vi "Send Cmd To Stimulator.vi"(0 "Stimulator":T1={"Stim Open Data"={"Name"="", "Mode"=enum."LIVE", "Visa Timeout"=0}, "Stim Init Data"={"Frequency"=0.0, "N Factor"=0, "D/T Int"=0.0, "Active Channels"=[FALSE], "LF Channels"=[]}, "Stim Update Data"={"Pulse Mode"=[], "Current"=[], "Pulse Dur"=[]}, "Stim Status"={"Open"=FALSE, "On"=FALSE}}, 1 "Command":T7, 3 "error in (no error)":errorcluster) -> (4 "Numeric Response":u8, 5 "Stimulator":T1={"Stim Open Data"={"Name"="", "Mode"=enum."LIVE", "Visa Timeout"=0}, "Stim Init Data"={"Frequency"=0.0, "N Factor"=0, "D/T Int"=0.0, "Active Channels"=[FALSE], "LF Channels"=[]}, "Stim Update Data"={"Pulse Mode"=[], "Current"=[], "Pulse Dur"=[]}, "Stim Status"={"Open"=FALSE, "On"=FALSE}}, 6 "Command":T7, 7 "Log Entry":string, 8 "error out":errorcluster)   [LabVIEW 2019]
uses:
  Data Type Defs/Stimulator.ctl
  Data Type Defs/Stim Open Data.ctl
  Data Type Defs/Stim Init Data.ctl
  Data Type Defs/Stim Update Data.ctl
  Data Type Defs/Pulse Mode (array).ctl
  Data Type Defs/Stim Status.ctl
  Bits Library/Get Bit (U8).vi
  Bits Library/Change Bit (U8).vi
  Bits Library/Bits.lvlib
panel:
  out "Write Error":errorcluster
  out "Bytes written":u32
  out "Bytes read":u32
  out "Read Error":errorcluster
  out "resulting string":string
  out "string":string
  out "hex integer string":string
  out "Number Out":u8 format="%.0x"
  out "appended array":bool[](array[boolean])
  out "element":u8 format="%0d"
  out "unsigned byte array 2":u8[](array[numeric]) format="%08b"
  out "Bytes available":u32
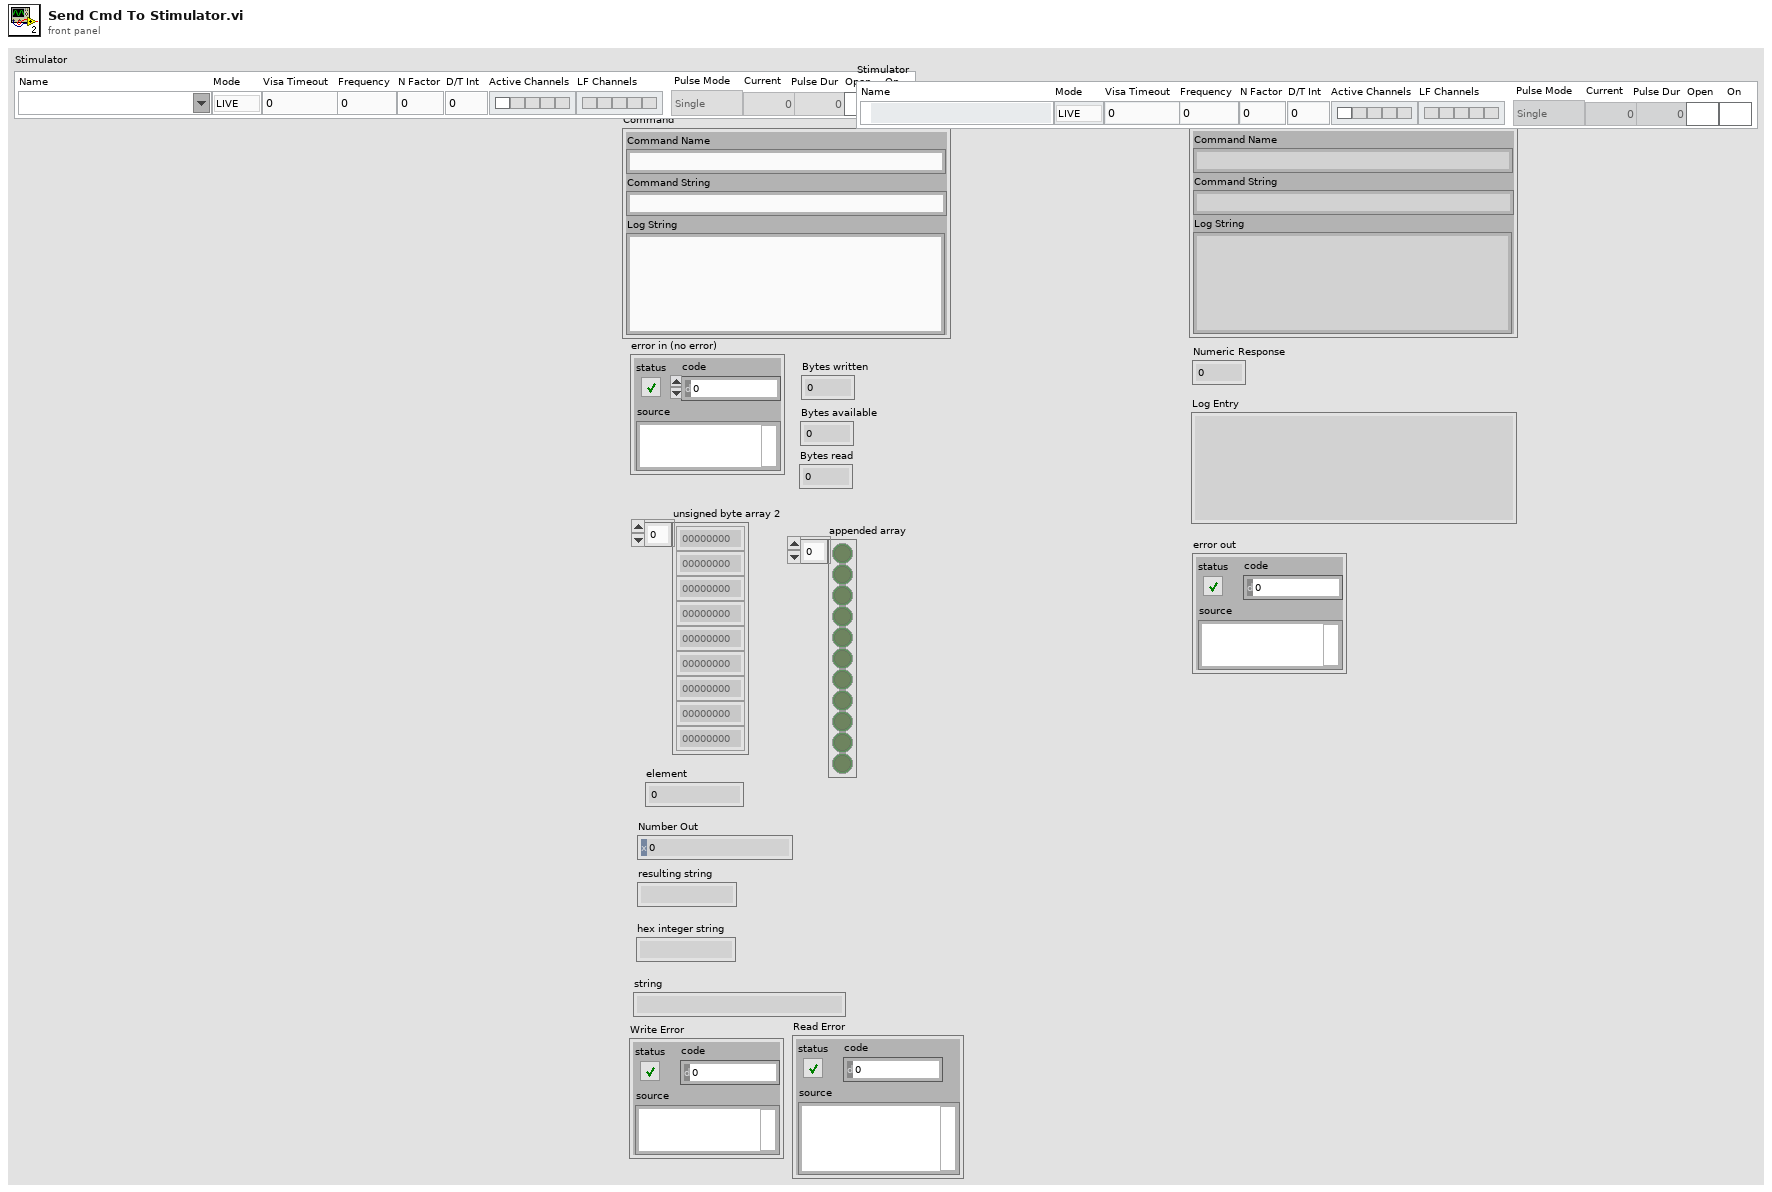
[diagram p1: front panel]
types:
  T1 = typedef "Stimulator.ctl" = cluster{"Stim Open Data":T2, "Stim Init Data":T3, "Stim Update Data":T4, "Stim Status":T6}
  T2 = typedef "Stim Open Data.ctl" = cluster{"Name":refnum<visa-resource-name>, "Mode":enum16{"LIVE", "SIM"}, "Visa Timeout":u32}
  T3 = typedef "Stim Init Data.ctl" = cluster{"Frequency":dbl, "N Factor":u8, "D/T Int":dbl, "Active Channels":bool[], "LF Channels":bool[]}
  T4 = typedef "Stim Update Data.ctl" = cluster{"Pulse Mode":T5, "Current":u32[], "Pulse Dur":u32[]}
  T5 = typedef "Pulse Mode (array).ctl" = enum16{"Single", "Doublet", "Triplet"}[]
  T6 = typedef "Stim Status.ctl" = cluster{"Open":bool, "On":bool}
  T7 = cluster{"Command Name":string, "Command String":string, "Log String":string}
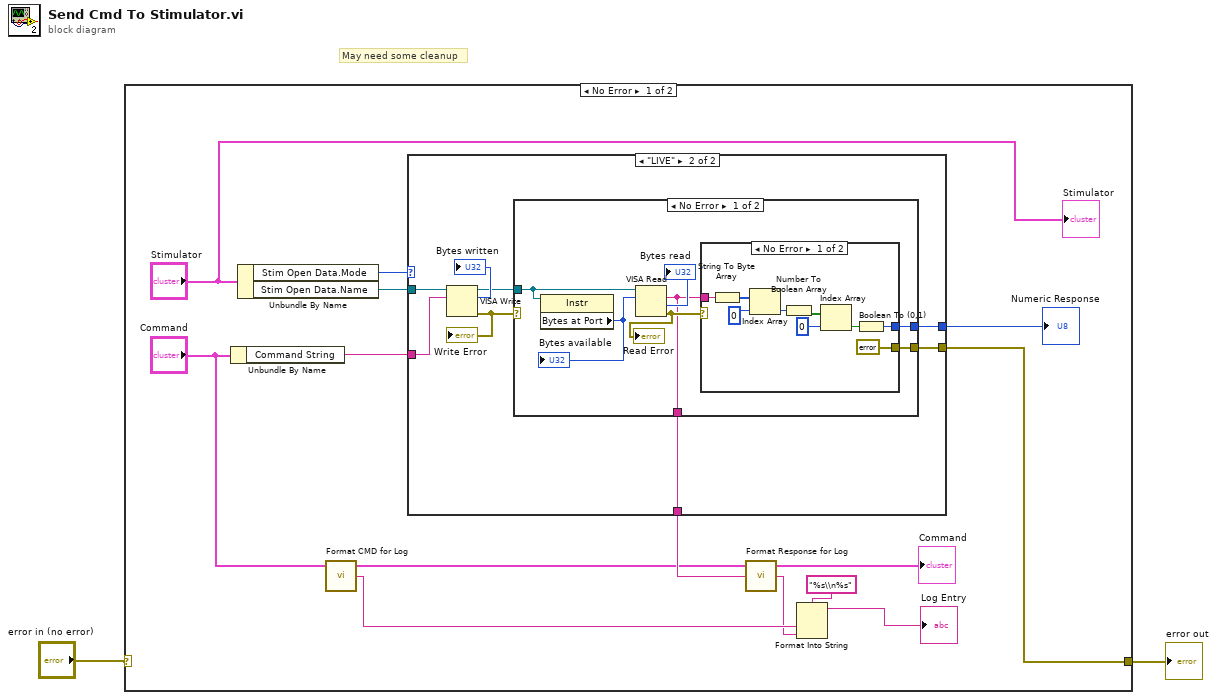
[diagram p0: block diagram]
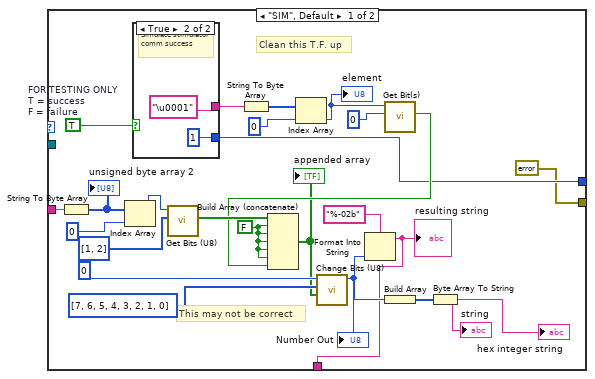
[diagram p2: hidden frame]
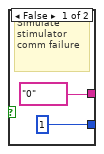
[diagram p3: hidden frame]
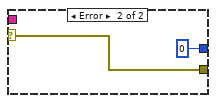
[diagram p4: hidden frame]
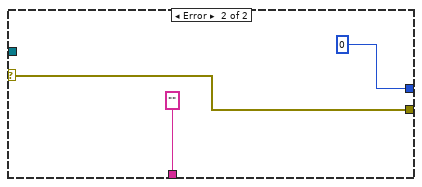
[diagram p5: hidden frame]
diagram:
  # "May need some cleanup"
  n1 = case shown="No Error" "error in (no error)" {
    selector: "error in (no error)" -> [_ w74]
    tunnel: [w12 w74] -> w1
    frame No Error {
      n2 = Unbundle By Name("Command") -> ("Command String"=w14:string)
      n3 = Unbundle By Name("Stimulator") -> ("Stim Open Data.Mode"=w16:enum16{"LIVE", "SIM"}, "Stim Open Data.Name"=w3:refnum<visa-resource-name>)
      n4 = call "Format CMD for Log.vi"("Command"="Command") -> ("Stim CMD for Log"=w8:string, "Command"=w10:T7)  [unwired: 2 in, 1 out]
      n5 = case shown="\"LIVE\"" w16 {
        tunnel: w14 -> [w39 w52]
        tunnel: [w19 w48] -> w13
        tunnel: [errorcluster {"status"=FALSE, "code"=0, "source"=""} ("error IO") w47] -> w12
        tunnel: [w18 w46] -> w11
        tunnel: w3 -> [_ w45]
        frame "SIM", Default {
          w30 = FALSE
          w40 = TRUE  # FOR TESTING ONLY T = success F = failure
          # "Clean this T.F. up"
          # "This may not be correct"
          n6 = String To Byte Array(string=w39) -> (unsigned byte array=w38:u8[])
          "unsigned byte array 2" <- w38
          n7 = Index Array(array=w38, index=0) -> (element=w36:u8)
          n8 = case shown="True" w40 {
            tunnel: ["0" "\u0001"] -> w32
            tunnel: [1 1] -> w19
            frame False {
              # "Simulate stimulator comm failure"
            }
            frame True {
              # "Simulate stimulator comm success"
            }
          }
          n9 = call "Get Bits (U8).vi"("Bits"=u8[] [1, 2], "Number"=w36) -> ("Values"=w31:bool[])  [unwired: 8 in, 1 out]
          n10 = String To Byte Array(string=w32) -> (unsigned byte array=w34:u8[])
          n11 = Index Array(array=w34, index=0) -> (element=w27:u8)
          "element" <- w27
          n12 = call-poly "Get Bit(s).vi"("Bit"=u8 0, "Number"=w27) -> ("Value"=w25:bool)  [unwired: 8 in, 1 out]
          n13 = Build Array (concatenate)(w31, w30, w30, w30, w30, w30, w25) -> (w21:bool[])
          "appended array" <- w21
          n14 = call "Change Bits (U8).vi"("Values"=w21, "Bits"=u8[] [7, 6, 5, 4, 3, 2, 1, 0], "Number"=u8 0) -> ("Number Out"=w20:u8)  [unwired: 8 in]
          "Number Out" <- w20
          n15 = Format Into String(format string="%-02b", w20) -> (resulting string=w18:string)  [unwired: 2 in, 1 out]
          "resulting string" <- w18
          n16 = Build Array(w20) -> (w24:u8[])
          n17 = Byte Array To String(unsigned byte array=w24) -> (string=→"hex integer string" →"string":string)
        }
        frame "LIVE" {
          n18 = VISA Write(VISA resource name=w45, write buffer=w52) -> (VISA resource name out=w49:refnum<visa-resource-name>, return count=→"Bytes written":u32, error out=w50:errorcluster)  [unwired: 1 in]
          "Write Error" <- w50
          n19 = case shown="No Error" w50 {
            selector: w50 -> [_ w73]
            tunnel: w49 -> [w58 _]
            tunnel: [w56 u8 0] -> w48
            tunnel: [w54 w73] -> w47
            tunnel: [w53 "" ("read buffer")] -> w46
            frame No Error {
              n20 = property class="Instr"(reference=w58) -> ("Bytes at Port"=w57:u32)  [unwired: 1 in, 2 out]
              "Bytes available" <- w57
              n21 = VISA Read(VISA resource name=w58, byte count=w57) -> (read buffer=w53:string, return count=→"Bytes read":u32, error out=w59:errorcluster)  [unwired: 1 in, 1 out]
              "Read Error" <- w59
              n22 = case shown="No Error" w59 {
                selector: w59 -> [_ w70]
                tunnel: [w60 u8 0] -> w56
                tunnel: w53 -> [w66 _]
                tunnel: [errorcluster {"status"=FALSE, "code"=0, "source"=""} ("error IO") w70] -> w54
                frame No Error {
                  n23 = String To Byte Array(string=w66) -> (unsigned byte array=w68:u8[])
                  n24 = Index Array(array=w68, index=0) -> (element=w64:u8)
                  n25 = Number To Boolean Array(number=w64) -> (Boolean array=w63:bool[])
                  n26 = Index Array(array=w63, index=0) -> (element=w61:bool)
                  n27 = Boolean To (0,1)(Boolean=w61) -> (0, 1=w60:i16)
                }
                frame Error {
                }
              }
            }
            frame Error {
            }
          }
        }
      }
      "Numeric Response" <- w13
      n28 = call "Format Response for Log.vi"("Response"=w11, "Command"=w10) -> ("Stim RSP for Log"=w5:string, "Command"=→"Command":T7)  [unwired: 1 in, 1 out]
      n29 = Format Into String(format string="%s\\n%s", w8, w5) -> (resulting string=→"Log Entry":string)  [unwired: 2 in, 1 out]
      "Stimulator" <- "Stimulator"
    }
    frame Error {
    }
  }
  "error out" <- w1
